vi "PH_Beckhoff_StepMot.Action Request Settings.vi"(0 "VI in":refnum<vi>, 5 "error in":errorcluster) -> (14 "VI out":refnum<vi>, 19 "error out":errorcluster)   [LabVIEW 2014, in "PH_Beckhoff_StepMot.lvlib"]
uses:
  PH_Beckhoff_StepMot.lvlib
  instr.lib/Beckhoff/Specials/Step Motor Klemmen/Beckhoff.Step Motor - Klemmen.ctl
  PH_Beckhoff_StepMot.Axis Cluster.ctl
  instr.lib/Beckhoff/Specials/Step Motor Klemmen/Beckhoff.Step Motor - Motor Configuration.ctl
  instr.lib/Beckhoff/Read and Write Register/Step Motor Klemmen/Beckhoff.Step Motor - Feature Register 1.ctl
  instr.lib/Beckhoff/Read and Write Register/Step Motor Klemmen/Beckhoff.Step Motor - Feature Register 2.ctl
  PH_Beckhoff/PH_Beckhoff.lvlib
  PH_Basics/PH_Stepmotor_BaseClass/PH_Stepmotor_BaseClass.lvlib
  instr.lib/Beckhoff/Beckhoff - Driver np.lvlib
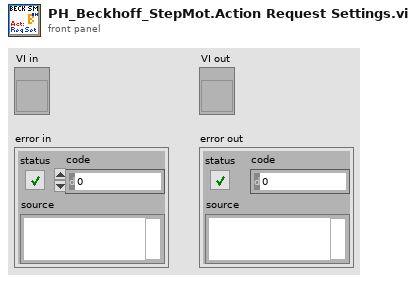
[diagram p1: front panel]
types:
  T1 = typedef "PH_Beckhoff_StepMot.lvlib/PH_Beckhoff_StepMot.i attribute.ctl" = cluster{"Axes Settings":T2[], "GUI Refs":cluster{"Axes Settings":refnum<vi>, "Stati":refnum<vi>}, "Get Beckhoff Settings":bool}
  T2 = typedef "PH_Beckhoff_StepMot.lvlib/PH_Beckhoff_StepMot.Axis Cluster.ctl" = cluster{"Step Motor Configuration":T3, "To set?":bool, "Endswitch inverted?":bool}
  T3 = typedef "Beckhoff - Driver np.lvlib/Beckhoff.Step Motor - Motor Configuration.ctl" = cluster{"Feature Register":T4, "I max A [mA]":dbl, "I max B [mA]":dbl, "v min":u32, "v max":u32, "a max":u32, "I hold [%]":u32, "Steps/qp":u32, "Feature Register 2":T5}
  T4 = typedef "Beckhoff - Driver np.lvlib/Beckhoff.Step Motor - Feature Register 1.ctl" = cluster{"en Auto Start":bool, "en Auto Stop":bool, "dis Wd Timer":bool, "OP Mode 1":bool, "OP Mode 2":bool, "Ramp Type":bool, "inv Pos Feedback":bool, "en User Cur Table":bool, "en Latch Evt Clr Pos":bool, "en Multi Latch Vals":bool, "en Sign Disp*":bool, "Feedback Type*":bool, "en neg Gate Lock*":bool, "en pos Gate Lock*":bool, "dis Enc Fltr*":bool, "en Counter Mode*":bool}
  T5 = typedef "Beckhoff - Driver np.lvlib/Beckhoff.Step Motor - Feature Register 2.ctl" = cluster{"rev Homing Dir":bool, "en Decac Ramp":bool, "Latch Reg Pos":bool, "Show Idle":bool, "dis Ref Input 1":bool, "dis Ref Input 2":bool, "en ext Auto Start":bool, "N/A":bool, "N/A":bool, "N/A":bool, "N/A":bool, "N/A":bool, "en Clr Proc Data":bool, "en Man Ecl Tolerce*":bool, "rev Dig Input 1":bool, "rev Dig Input 2":bool}
  T6 = typedef "Beckhoff - Driver np.lvlib/Beckhoff.Step Motor - Klemmen.ctl" = enum16{"none", "KL 2531", "KL 2541"}
  T7 = typedef "PH_Beckhoff.lvlib/PH_Beckhoff.i attribute.ctl" = cluster{"GUI Refs":T8, "operation?":bool, "Default Prdc Interval":i32, "Connection":T9, "AMS Net ID":T10, "Klemmencluster: # of":T11, "Values":T12, "IP":string, "Description":string, "configured?":bool, "Change Manager":cluster{"Detemination wanted?":bool, "Values changed at":cluster{"Sonderklemmen Inputs":i32[], "Analog Inputs":i32[], "Analog Outputs":i32[], "Digital Inputs":i32[], "Digital Outputs":i32[]}}, "Difference to handle an analog input as change":u32}
  T8 = typedef "PH_Beckhoff.lvlib/PH_Beckhoff.GUI Refs.ctl" = cluster{"ADS Error":refnum<vi>, "Values":refnum<vi>, "configured?":refnum<vi>, "Connection":refnum<vi>, "IP":refnum<vi>, "Prdc Int [ms]":refnum<vi>}
  T9 = typedef "PH_Beckhoff.lvlib/PH_Beckhoff.Connectivity.ctl" = cluster{"DLL?":bool, "Port?":bool, "Client?":bool, "Ping?":bool, "unsuccessful Pings":u32}
  T10 = typedef "Beckhoff - Driver np.lvlib/Beckhoff Access.ctl" = cluster{"DLL path":path, "AMS Net ID":cluster{"1st # of IP":u8, "2nd # of IP":u8, "3rd # of IP":u8, "4th # of IP":u8, "In Port":u8, "Out Port":u8}}
  T11 = typedef "Beckhoff - Driver np.lvlib/Klemmendeclarer.ctl" = cluster{"Offset due to Sonderklemms":u32, "analog Inputs":u32, "analog Outputs":u32, "digital Input Bits":u32, "digital Output Bits":u32}
  T12 = typedef "PH_Beckhoff.lvlib/PH_Beckhoff.Values.ctl" = cluster{"Sonderklemmen Inputs":T13, "Analog Inputs":T14, "Analog Outputs":T16, "Digital Inputs":T17, "Digital Outputs":T18}
  T13 = typedef "PH_Beckhoff.lvlib/PH_Beckhoff.Sonderklemmen Inputs.ctl" = cluster{"Total Length":u32, "Name":string, "Value":u64, "Quality":bool, "Service ID":i32, "Offset":u32, "Length":u32}[]
  T14 = typedef "PH_Beckhoff.lvlib/PH_Beckhoff.Analog Inputs.ctl" = cluster{"Name":string, "Value":u32, "Quality":bool, "Service ID":i32, "Sca Type":T15}[]
  T15 = typedef "PH_Beckhoff.lvlib/PH_Beckhoff.Scaling Type.ctl" = enum16{"none", "0 ... 15 Bit -> 0 ... 5", "0 ... 15 Bit -> 0 ... 10", "0 ... 15 Bit -> 0 ... 25", "0 ... 15 Bit -> 4 ... 20", "0 ... 15 Bit -> 0 ... 1", "0 ... 15 Bit -> 0 ... 20000", "0 ... 15 Bit -> 0 ... 24000"}
  T16 = typedef "PH_Beckhoff.lvlib/PH_Beckhoff.Analog Outputs.ctl" = cluster{"Name":string, "Value":u32, "Quality":bool, "Wanted Value":u32, "Service ID":i32, "Sca Type":T15}[]
  T17 = typedef "PH_Beckhoff.lvlib/PH_Beckhoff.Digital Inputs.ctl" = cluster{"Name":string, "Value":bool, "Quality":bool, "Service ID":i32, "inverted?":bool}[]
  T18 = typedef "PH_Beckhoff.lvlib/PH_Beckhoff.Digital Outputs.ctl" = cluster{"Name":string, "Value":bool, "Quality":bool, "Wanted Value":bool, "Service ID":i32, "inverted?":bool}[]
  T19 = typedef "PH_Stepmotor_BaseClass.lvlib/PH_Stepmotor_BaseClass.i attribute.ctl" = cluster{"Device Error":errorcluster, "Axes PSDB Thread":cluster{"Ref":refnum<vi>, "Q-Ref":refnum<queue>, "Data Status":T20}, "Axes":T21[], "Axes PSDB Infos":cluster{"GUI Name":string, "PSDB Instance ID":i32, "PSDB Status Service ID":i32, "Axis":i32, "Class":string}[], "GUI Refs":T26}
  T20 = typedef "PH_PSDBWriter.lvlib/PH_PSDBWriter.Data Status.ctl" = i16
  T21 = typedef "PH_Stepmotor_BaseClass.lvlib/PH_Stepmotor_BaseClass.Axis Attributes.ctl" = cluster{"Settings":T22, "Endswitch?":bool, "DIM Service IDs":T24, "Activity":T25, "Configured?":bool, "Position":cluster{"Current":i32, "Target":i32}, "Position to set":cluster{"New?":bool, "Wanted":i32}, "Stop?":bool, "Reset?":bool, "Move?":bool, "Nothing connected?":bool}
  T22 = typedef "PH_Stepmotor_BaseClass.lvlib/PH_Stepmotor_BaseClass.Axis Settings.ctl" = cluster{"Sign change":bool, "Width":dbl, "Calibration":dbl, "Unit":string, "Motor Type":T23, "Unit Width":string, "Unit CF":string}
  T23 = typedef "PH_Stepmotor_BaseClass.lvlib/PH_Stepmotor_BaseClass.Motor Type.ctl" = enum16{"Unspecific", "OWIS 49.120.2633", "OWIS 49.060.1033", "OWIS 43.040.2558", "Diamond Motion 2200 series", "OWIS 49.120.266B.MV6", "Calorimeter", "Linear Stage 1", "MICOS VT-80", "MICOS VT-80 S", "Standa Rotstage nt0.95A", "PUF RA 320.200", "PUF RA 800.200", "PUF RA 800.400", "PUF RA 400.50", "1324.nn.800.50", "1324.n9c.800.50", "1324.nn.320.200", "1324.nn.400.200", "1324.nn.800.200", "1324.nn.400.50", "1324.8c9c.800.50", "1324.8c9c.400.200"}
  T24 = typedef "PH_Stepmotor_BaseClass.lvlib/PH_Stepmotor_BaseClass.Axis DIM Service IDs.ctl" = cluster{"Settings":i32, "Information":i32}
  T25 = typedef "PH_Stepmotor_BaseClass.lvlib/PH_Stepmotor_BaseClass.Axis Activity.ctl" = enum16{"No Information", "stopped", "running", "Failure", "Alarm", "stopped at backward ES", "stopped at foreward ES"}
  T26 = typedef "PH_Stepmotor_BaseClass.lvlib/PH_Stepmotor_BaseClass.GUI Refs.ctl" = cluster{"Axes Configuration":refnum<vi>, "Device Error":refnum<vi>, "Axes PSDB Infos":refnum<vi>}
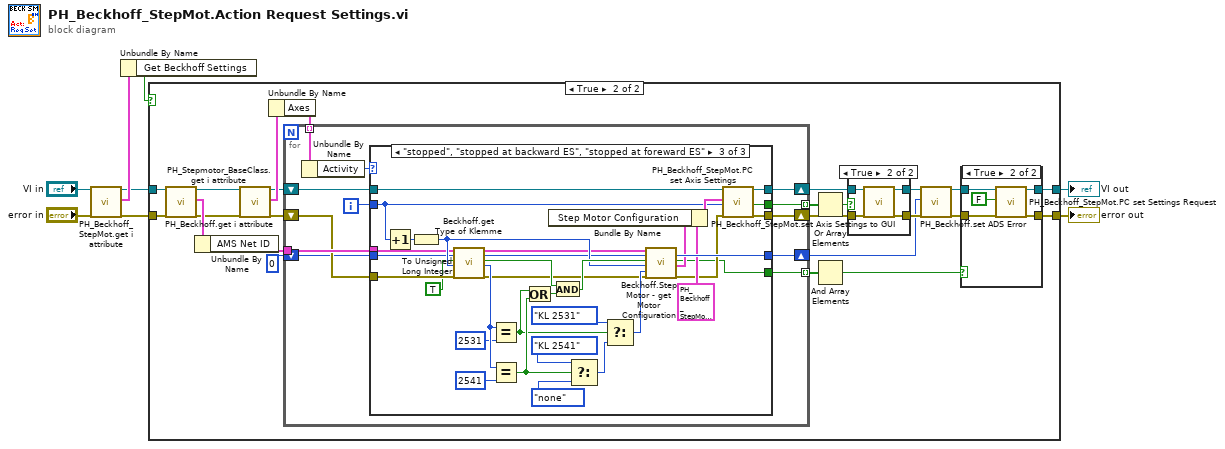
[diagram p0: block diagram]
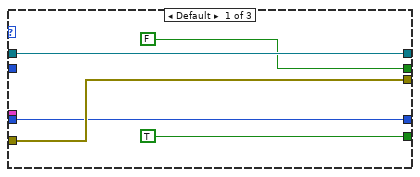
[diagram p5: hidden frame]
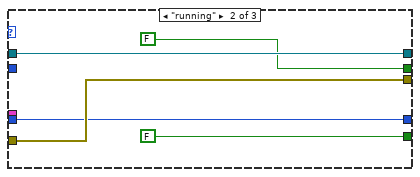
[diagram p6: hidden frame]
diagram:
  n1 = call "PH_Beckhoff_StepMot.get i attribute.vi"("i ref in"="VI in", "error in (no error)"="error in") -> ("i ref out"=w7:refnum<vi>, "i attribute"=w8:T1, "error out"=w6:errorcluster)  [unwired: 15 in]
  n2 = Unbundle By Name(w8) -> ("Get Beckhoff Settings"=w5:bool)
  n3 = case shown="True" w5 {
    tunnel: w7 -> [w10 w19]
    tunnel: w6 -> [w9 w18]
    tunnel: [w10 w12] -> w2
    tunnel: [w9 w11] -> w1
    frame False {
    }
    frame True {
      n4 = call "PH_Beckhoff.get i attribute.vi"("i ref in"=w19, "error in (no error)"=w18) -> ("i ref out"=w17:refnum<vi>, "i attribute"=w34:T7, "error out"=w16:errorcluster)  [unwired: 15 in]
      n5 = Unbundle By Name(w34) -> ("AMS Net ID"=w33:T10)
      n6 = call "PH_Stepmotor_BaseClass.get i attribute.vi"("i ref in"=w17, "error in (no error)"=w16) -> ("i ref out"=w15:refnum<vi>, "i attribute"=w22:T19, "error out"=w14:errorcluster)  [unwired: 15 in]
      n7 = Unbundle By Name(w22) -> ("Axes"=w21:T21[])
      n8 = for {
        tunnel: w33 -> [w59]
        shift-right: [w55] -> w29
        shift-left: w14 -> [w58]
        shift-right: [w56] -> w20
        shift-left: 0 ("ADS Error out") -> [w57]
        shift-right: [w53] -> w26
        shift-left: w15 -> [w54]
        tunnel: [w48] -> w32 mode=indexing
        tunnel: [w52] -> w24 mode=indexing
        tunnel: w21 -> [w51] mode=indexing
        i -> [w50]
        n9 = Unbundle By Name(w51) -> ("Activity"=w49:T25)
        n10 = case shown="\"stopped\", \"stopped at backward ES\", \"stopped at foreward ES\"" w49 {
          tunnel: w59 -> [_ _ w85]
          tunnel: w58 -> [w63 w68 w88]
          tunnel: w57 -> [w61 w66 w84]
          tunnel: [w61 w66 w81] -> w56
          tunnel: [w63 w68 w76] -> w55
          tunnel: w54 -> [w64 w69 w74]
          tunnel: [w64 w69 w75] -> w53
          tunnel: [TRUE FALSE w71] -> w48
          tunnel: w50 -> [_ _ w73]
          tunnel: [FALSE ("Settings changed?") FALSE ("Settings changed?") w72] -> w52
          frame Default {
          }
          frame "running" {
          }
          frame "stopped", "stopped at backward ES", "stopped at foreward ES" {
            n11 = Increment(x=w73) -> (x+1=w102:i32)
            n12 = To Unsigned Long Integer(number=w102) -> (unsigned 32bit integer=w87:u32)
            n13 = call "Beckhoff.get Type of Klemme.vi"("AMS Net ID in"=w85, "ADS Error in (0)"=w84, "Read?"=TRUE, "# of Klemme [1 ...]"=w87, "error in"=w88) -> ("AMS Net ID out"=w83:T10, "ADS Error out"=w82:i32, "Read successful?"=w91:bool, "Klemmentyp"=w95:u32, "error out"=w86:errorcluster)  [unwired: 10 in]
            n14 = Equal?(x=w95, y=u32 2531) -> (x = y?=w97:bool)
            n15 = Equal?(x=w95, y=u32 2541) -> (x = y?=w98:bool)
            n16 = Or(x=w97, y=w98) -> (x .or. y?=w96:bool)
            n17 = And(x=w91, y=w96) -> (x .and. y?=w89:bool)
            n18 = Select(t=Beckhoff.Step_Motor_-_Klemmen."KL 2541" ("Klemme found 2"), s=w98, f=Beckhoff.Step_Motor_-_Klemmen."none") -> (s? t:f=w99:T6)
            n19 = Select(t=Beckhoff.Step_Motor_-_Klemmen."KL 2531" ("Klemme found 2"), s=w97, f=w99) -> (s? t:f=w90:T6)
            n20 = call "Beckhoff.Step Motor - get Motor Configuration.vi"("AMS Net ID in"=w83, "ADS Error in"=w82, "Read?"=w89, "# of Klemme [1 ...]"=w87, "Klemmentype"=w90, "error in (no error)"=w86) -> ("ADS Error out"=w81:i32, "Operation successful?"=w71:bool, "current Step Motor Configuration"=w78:T3, "error out"=w77:errorcluster)  [unwired: 9 in, 1 out]
            n21 = Bundle By Name(cluster=T2 {"Step Motor Configuration"={"Feature Register"={"en Auto Start"=FALSE, "en Auto Stop"=FALSE, "dis Wd Timer"=FALSE, "OP Mode 1"=FALSE, "OP Mode 2"=FALSE, "Ramp Type"=FALSE, "inv Pos Feedback"=FALSE, "en User Cur Table"=FALSE, "en Latch Evt Clr Pos"=FALSE, "en Multi Latch Vals"=FALSE, "en Sign Disp*"=FALSE, "Feedback Type*"=FALSE, "en neg Gate Lock*"=FALSE, "en pos Gate Lock*"=FALSE, "dis Enc Fltr*"=FALSE, "en Counter Mode*"=FALSE}, "I max A [mA]"=0.0, "I max B [mA]"=0.0, "v min"=0, "v max"=0, "a max"=0, "I hold [%]"=0, "Steps/qp"=0, "Feature Register 2"={"rev Homing Dir"=FALSE, "en Decac Ramp"=FALSE, "Latch Reg Pos"=FALSE, "Show Idle"=FALSE, "dis Ref Input 1"=FALSE, "dis Ref Input 2"=FALSE, "en ext Auto Start"=FALSE, "N/A"=FALSE, "N/A"=FALSE, "N/A"=FALSE, "N/A"=FALSE, "N/A"=FALSE, "en Clr Proc Data"=FALSE, "en Man Ecl Tolerce*"=FALSE, "rev Dig Input 1"=FALSE, "rev Dig Input 2"=FALSE}}, "To set?"=FALSE, "Endswitch inverted?"=FALSE} ("Axis Settings"), "Step Motor Configuration"=w78) -> (w79:T2)
            n22 = call "PH_Beckhoff_StepMot.PC set Axis Settings.vi"("VI in"=w74, "Axis Settings"=w79, "Axis"=w73, "error in (no error)"=w77) -> ("VI out"=w75:refnum<vi>, "Settings changed?"=w72:bool, "error out"=w76:errorcluster)  [unwired: 13 in]
          }
        }
      }
      n23 = Or Array Elements(Boolean array=w24) -> (logical OR=w23:bool)
      n24 = And Array Elements(Boolean array=w32) -> (logical AND=w13:bool)
      n25 = case shown="True" w23 {
        tunnel: w29 -> [w42 w47]
        tunnel: [w42 w46] -> w27
        tunnel: w26 -> [w43 w45]
        tunnel: [w43 w44] -> w25
        frame False {
        }
        frame True {
          n26 = call "PH_Beckhoff_StepMot.set Axis Settings to GUI.vi"("VI in"=w45, "error in (no error)"=w47) -> ("VI out"=w44:refnum<vi>, "error out"=w46:errorcluster)  [unwired: 16 in]
        }
      }
      n27 = call "PH_Beckhoff.set ADS Error.vi"("i ref in"=w25, "ADS Error"=w20, "error in"=w27) -> ("i ref out"=w30:refnum<vi>, "error out"=w28:errorcluster)  [unwired: 15 in]
      n28 = case shown="True" w13 {
        tunnel: w30 -> [w36 w41]
        tunnel: w28 -> [w35 w40]
        tunnel: [w36 w39] -> w12
        tunnel: [w35 w38] -> w11
        frame False {
        }
        frame True {
          n29 = call "PH_Beckhoff_StepMot.PC set Settings Request.vi"("VI in"=w41, "Get Beckhoff Settings"=FALSE, "error in (no error)"=w40) -> ("VI out"=w39:refnum<vi>, "error out"=w38:errorcluster)  [unwired: 15 in]
        }
      }
    }
  }
  "error out" <- w1
  "VI out" <- w2
